vi "BaseTemplate_4x4x4_Create.vi"(8 "Error In":errorcluster, 11 "reference in":refnum<class "BaseTemplate_4x4x4.lvclass">) -> (0 "Error Out":errorcluster, 3 "reference out":refnum<class "BaseTemplate_4x4x4.lvclass">)   [LabVIEW 2020, in "BaseTemplate_4x4x4.lvclass"]
uses:
  <resource>/Framework/Providers/Open_GDS/ClassProviders/Provider_EndevoGOOP300/Templates/BaseTemplate_4x4x4/BaseTemplate_4x4x4.lvclass
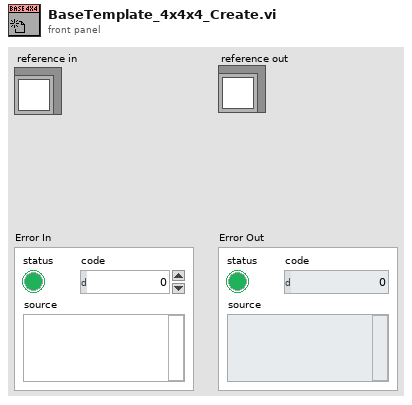
[diagram p1: front panel]
types:
  T1 = typedef "BaseTemplate_4x4x4.lvclass/ObjectAttributes.ctl" = cluster{"Attribute1":dbl}
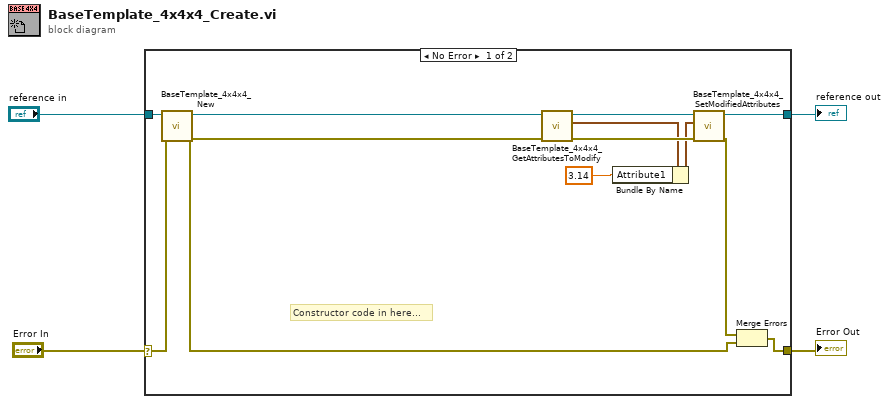
[diagram p0: block diagram]
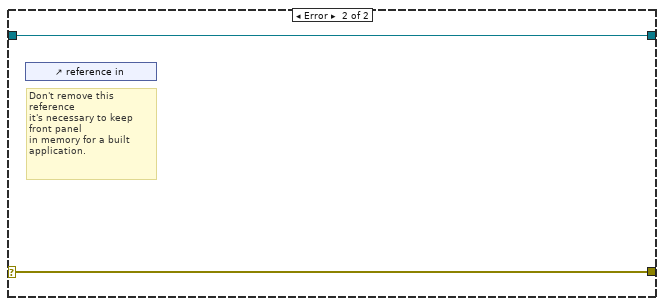
[diagram p2: hidden frame]
diagram:
  n1 = case shown="No Error" "Error In" {
    selector: "Error In" -> [w16 w18]
    tunnel: [w7 w18] -> w4
    tunnel: "reference in" -> [w9 w17]
    tunnel: [w10 w17] -> w2
    frame No Error {
      # "Constructor code in here..."
      n2 = call <resource>:"BaseTemplate_4x4x4_New.vi"("error in (no error)"=w16, "reference in"=w9) -> ("error out"=w5:errorcluster, "reference out"=w8:refnum<class "BaseTemplate_4x4x4.lvclass">)  [unwired: 6 in, 2 out]
      n3 = call <resource>:"BaseTemplate_4x4x4_GetAttributesToModify.vi"("error in (no error)"=w5, "reference in"=w8) -> ("error out"=w15:errorcluster, "Attributes"=w13:T1, "reference out"=w14:refnum<class "BaseTemplate_4x4x4.lvclass">)  [unwired: 6 in, 1 out]
      n4 = Bundle By Name(cluster=w13, "Attribute1"=3.14 ("attribute1")) -> (w12:T1)
      n5 = call <resource>:"BaseTemplate_4x4x4_SetModifiedAttributes.vi"("error in (no error)"=w15, "Attributes"=w12, "reference in"=w14) -> ("error out"=w6:errorcluster, "reference out"=w10:refnum<class "BaseTemplate_4x4x4.lvclass">)  [unwired: 7 in]
      n6 = Merge Errors(w6, w5) -> (w7:errorcluster)
    }
    frame Error {
      # "Don't remove this reference\nit's necessary to keep front panel\nin memory for a built application."
      n7 = control-ref of="reference in"() -> ()  [unwired: 1 out]
    }
  }
  "Error Out" <- w4
  "reference out" <- w2
